vi "Collapse Tree.vi"(8 "error in (no error)":errorcluster, 11 "Tree Ref in":refnum<vi>) -> (0 "error out":errorcluster, 3 "Tree Ref out":refnum<vi>)   [LabVIEW 2017, in "Report Viewer.lvlib"]
uses:
  Report Viewer.lvlib
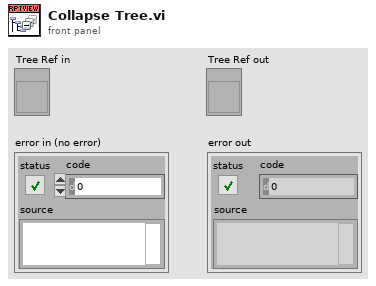
[diagram p1: front panel]
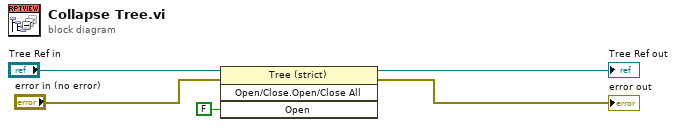
[diagram p0: block diagram]
diagram:
  n1 = invoke class="Tree (strict)" method="Open/Close.Open/Close All"(reference="Tree Ref in", error in="error in (no error)", "Open"=FALSE ("Open?")) -> (reference out=→"Tree Ref out":refnum<vi>, error out=→"error out":errorcluster)  [unwired: 1 in, 2 out]
